vi "GetGroupIdLookupKey.vi"(10 "Properties":T1[](array[typedef]), 11 "AssetNodeId":string) -> (3 "group id lookup key":string)   [LabVIEW 2017, in "Trigger.lvlib"]
uses:
  <vilib>/addons/InsightCM/Devices/Shared/Common/Trigger/Trigger.lvlib
  <vilib>/addons/InsightCM/MessageBus/Base/controls/KeyValuePair.ctl
  <vilib>/addons/InsightCM/Utilities/PropertyHelpers/PropertyHelpers.lvlib
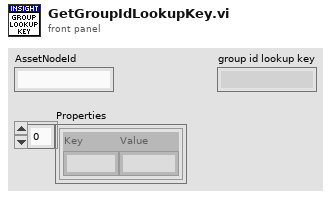
[diagram p1: front panel]
types:
  T1 = typedef "KeyValuePair.ctl" = cluster{"Key":string, "Value":string}
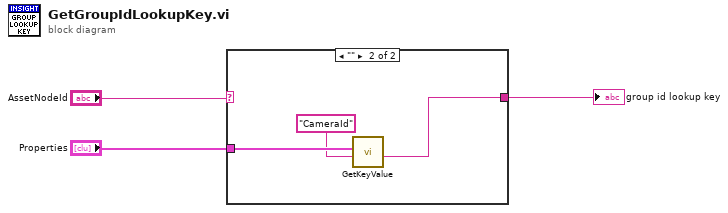
[diagram p0: block diagram]
diagram:
  n1 = case shown="\"\"" "AssetNodeId" {
    selector: "AssetNodeId" -> [w4 _]
    tunnel: "Properties" -> [_ w7]
    tunnel: [w4 w5] -> w3
    frame Default {
    }
    frame "" {
      n2 = call <vilib>:"GetKeyValue.vi"("key"="CameraId", "key value pairs"=w7) -> ("value"=w5:string)  [unwired: 7 in, 2 out]
    }
  }
  "group id lookup key" <- w3
